vi "关于.vi"() -> ()   [LabVIEW 8.6]
panel:
  out "信息显示":string
  in  "?":bool
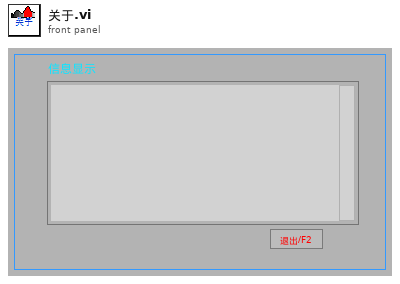
[diagram p1: front panel]
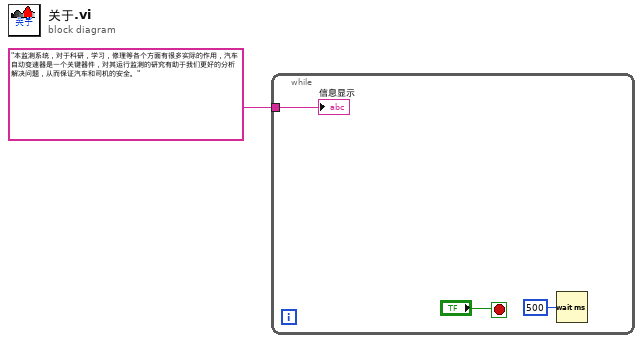
[diagram p0: block diagram]
diagram:
  n1 = while {
    tunnel: "本监测系统，对于科研，学习，修理等各个方面有很多实际的作用，汽车自动变速器是一个关键器件，对其运行监测的研究有助于我们更好的分析解决问题，从而保证汽车和司机的安全。" -> [w2]
    stop <- "?" stop-if-true
    n2 = Wait (ms)(milliseconds to wait=u32 500 ("等待时间（毫秒）")) -> ()  [unwired: 1 out]
    "信息显示" <- w2
  }
